vi "Lab Panel V5.22.1.vi"() -> ()   [LabVIEW 2013] (continued)
                      frame #1 {
                        n566 = local read "DISP LAB01-2"() -> (w843:T4)
                        n567 = stacked-sequence {
                          tunnel: "LAB01-2" -> [w845 w847]
                          frame #0 {
                            n568 = call "sub vi - defrag tdms v1.vi"("panel id"=w845) -> ("error out"=w844:errorcluster)  [unwired: 10 in]
                            n569 = local write "data file error"(w844) -> ()
                          }
                          frame #1 {
                            n570 = call "Save data file (stop) v3.vi"("panel id"=w847) -> ("network file save error"=w846:errorcluster)  [unwired: 9 in, 1 out]
                            n571 = local write "RESULT LAB01-2"(FALSE) -> ()
                            n572 = local write "data file error"(w846) -> ()
                          }
                        }
                        n573 = Bundle(cluster=w843, "STATUS"="STOP") -> (w841:T4)  [unwired: 2 in]
                        n574 = local write "DISP LAB01-2"(w841) -> ()
                      }
                    }
                  }
                  frame True {
                    n575 = local read "SIG LAB01-2"() -> (w850:T2)
                    n576 = stacked-sequence {
                      seq-local: [w861 _] -> [_ w865]
                      tunnel: w859 -> [_ w875]
                      tunnel: w858 -> [_ w874]
                      tunnel: w857 -> [_ w873]
                      tunnel: w856 -> [_ w872]
                      tunnel: w855 -> [_ w871]
                      tunnel: [_ w870] -> w854
                      tunnel: w853 -> [_ w869]
                      tunnel: w852 -> [_ w868]
                      tunnel: w851 -> [_ w867]
                      tunnel: w850 -> [w860 w866]
                      tunnel: w849 -> [_ w864]
                      frame #0 {
                        n577 = Unbundle(w860) -> ("AMPS"=w863:dbl)  [unwired: 4 out]
                        n578 = call "Check For Amps on v1.vi"("ID"="LAB01-2", "amps"=w863) -> ("amps"=w861:bool)  [unwired: 9 in]
                      }
                      frame #1 {
                        n579 = case shown="True" w865 {
                          tunnel: w875 -> [_ w888]
                          tunnel: w874 -> [_ w887]
                          tunnel: w873 -> [_ w886]
                          tunnel: w872 -> [_ w885]
                          tunnel: w871 -> [_ w884]
                          tunnel: [errorcluster {"status"=FALSE, "code"=0, "source"=""} ("error out") w883] -> w870
                          tunnel: w869 -> [_ w882]
                          tunnel: w868 -> [_ w881]
                          tunnel: w867 -> [_ w880]
                          tunnel: w866 -> [_ w879]
                          tunnel: w864 -> [_ w878]
                          frame False {
                            w876 = FALSE
                            n580 = local write "RUN LAB01-2"(w876) -> ()
                            n581 = local write "run lab01-2"(w876) -> ()
                          }
                          frame True {
                            n582 = stacked-sequence {
                              seq-local: [w889 _ _ _ _] -> [_ w913 _ _ _]
                              tunnel: w888 -> [w894 _ _ _ _]
                              tunnel: w887 -> [w891 _ _ _ _]
                              tunnel: w886 -> [w904 _ _ _ _]
                              tunnel: w885 -> [w897 _ _ _ _]
                              tunnel: w884 -> [w892 _ _ _ _]
                              tunnel: [_ w908 _ _ _] -> w883
                              tunnel: w882 -> [_ _ _ w935 _]
                              tunnel: w881 -> [_ _ _ w934 _]
                              tunnel: w880 -> [_ _ _ w933 _]
                              tunnel: w879 -> [_ _ _ _ _]
                              tunnel: w878 -> [_ _ _ _ w948]
                              frame #0 {
                                w890 = "\\"
                                n583 = local read "SET LAB01-2"() -> (w899:T5)
                                n584 = case shown="\"CYCLE TEST\"" w904 {
                                tunnel: ["L01-2-CHART TEST-" "L01-2-CYCLE TEST-" "L01-2-T-RISE TEST-"] -> w900
                                frame "CHART TEST", Default {
                                }
                                frame "CYCLE TEST" {
                                }
                                frame "T-RISE TEST" {
                                }
                                }
                                n585 = Unbundle(w899) -> ("DESCRIPTION"=w898:string)  [unwired: 4 out]
                                n586 = Concatenate Strings(w894, "\\", w892, w890, w891, w890) -> (w901:string)
                                n587 = String To Path(string=w901) -> (path=w903:path)
                                n588 = Concatenate Strings(w901, w900, w898, "-", w897, ".tdms") -> (w889:string)
                                n589 = Create Folder(path (use dialog)=w903) -> (error out=w902:errorcluster)  [unwired: 2 in, 2 out]
                                n590 = call <vilib>:"Clear Errors.vi"("error in (no error)"=w902) -> ()  [unwired: 6 in, 1 out]
                                n591 = global write "Global 1.vi" "LAB01-2 FILE"(w889) -> ()
                              }
                              frame #1 {
                                (unwired) FALSE
                                n592 = String To Path(string=w913) -> (path=w909:path)
                                n593 = TDMS Open(6:FALSE, 10:T21."create or replace" ("operation (0:open)"), 11:w909) -> (0:w908:errorcluster, 3:→"TDMS LAB01-2":refnum<k34>)  [unwired: 4 in]
                              }
                              frame #2 {
                                n594 = local read "SET LAB01-2"() -> (w919:T5)
                                n595 = local read "TDMS LAB01-2"() -> (w930:refnum<k34>)
                                n596 = Build Array("Testers Name", "Description", "Set Test Cycles", "T-Rise minutes", "T-Rise Deg C") -> (w920:string[])
                                n597 = Unbundle(w919) -> ("NAME"=w918:string, "DESCRIPTION"=w917:string, "CYCLES"=w916:dbl, "T-RISE mins"=w915:dbl, "T-RISE deg C"=w914:dbl)
                                n598 = Number To Decimal String(number=w916) -> (decimal integer string=w929:string)  [unwired: 1 in]
                                n599 = Number To Decimal String(number=w915) -> (decimal integer string=w928:string)  [unwired: 1 in]
                                n600 = Number To Decimal String(number=w914) -> (decimal integer string=w927:string)  [unwired: 1 in]
                                n601 = Build Array(w918, w917, w929, w928, w927) -> (w926:string[])
                                n602 = TDMS Set Properties(5:w926, 7:w920, 11:w930) -> ()  [unwired: 3 in, 4 out]
                              }
                              frame #3 {
                                n603 = local read "DISP LAB01-2"() -> (w932:T4)
                                n604 = Concatenate Strings("LAB01-2  ", w935) -> (w936:string)
                                n605 = Two Button Dialog(message=w936, 1:w933, 2:w934) -> (T button?=w938:bool)
                                n606 = case shown="True" w938 {
                                tunnel: w932 -> [w945 w946]
                                tunnel: [w945 w946] -> w942
                                tunnel: [w944 w947] -> w941
                                tunnel: [w943 w947] -> w940
                                frame False {
                                n607 = Unbundle(w945) -> ("CYCLE"=w944:dbl, "MINS"=w943:dbl)  [unwired: 1 out]
                                }
                                frame True {
                                w947 = 0.0
                                }
                                }
                                n608 = Bundle(cluster=w942, "CYCLE"=w941, "MINS"=w940, "STATUS"="RUN") -> (w931:T4)
                                n609 = local write "DISP LAB01-2"(w931) -> ()
                              }
                              frame #4 {
                                n610 = local read "TEMP START LAB01-2"() -> (w950:cluster{"TL":dbl, "TN":dbl})
                                n611 = Bundle(cluster=w950, "TL"=w948, "TN"=w948) -> (w949:cluster{"TL":dbl, "TN":dbl})
                                n612 = local write "TEMP START LAB01-2"(w949) -> ()
                              }
                            }
                          }
                        }
                      }
                    }
                  }
                }
              }
              event "RUN LAB02-1": Value Change {
                n613 = event-data() -> ("NewVal"=w956:bool)  [unwired: 1 in, 5 out]
                n614 = local read "SIG LAB02-1"() -> (w952:T2)
                n615 = case shown="True" w956 {
                  tunnel: w962 -> [_ w1000]
                  tunnel: w961 -> [_ w999]
                  tunnel: w959 -> [w964 w998]
                  tunnel: w960 -> [_ w997]
                  tunnel: w958 -> [_ w996]
                  tunnel: [w963 w995] -> w957
                  tunnel: w955 -> [_ w994]
                  tunnel: w954 -> [_ w993]
                  tunnel: w953 -> [_ w992]
                  tunnel: w952 -> [_ w991]
                  tunnel: w951 -> [_ w990]
                  frame False {
                    # "stop test"
                    n616 = stacked-sequence {
                      tunnel: w964 -> [w973 _]
                      tunnel: [w965 _] -> w963
                      frame #0 {
                        n617 = local read "DISP LAB02-1"() -> (w972:T4)
                        n618 = Unbundle(w972) -> ("CYCLE"=w970:dbl, "MINS"=w971:dbl)  [unwired: 1 out]
                        n619 = case shown="\"CYCLE TEST\"" w973 {
                          tunnel: w971 -> [_ _ w980]
                          tunnel: w970 -> [w978 w979 _]
                          tunnel: [w978 w979 w980] -> w969
                          frame "CHART TEST", Default {
                          }
                          frame "CYCLE TEST" {
                          }
                          frame "T-RISE TEST" {
                          }
                        }
                        n620 = local read "TDMS LAB02-1"() -> (w977:refnum<k34>)
                        n621 = Build Array("STOPPED") -> (w974:string[])
                        n622 = Build Array(w969) -> (w968:dbl[])
                        n623 = TDMS Write(0:w977, 5:"TEST RESULT", 7:w974, 9:w968) -> (4:w966:refnum<k34>, 15:w967:errorcluster)  [unwired: 2 in, 2 out]
                        n624 = TDMS Close(8:w967, 11:w966) -> (0:w965:errorcluster)  [unwired: 1 out]
                      }
                      frame #1 {
                        n625 = local read "DISP LAB02-1"() -> (w984:T4)
                        n626 = stacked-sequence {
                          tunnel: "LAB02-1" -> [w986 w988]
                          frame #0 {
                            n627 = call "sub vi - defrag tdms v1.vi"("panel id"=w986) -> ("error out"=w985:errorcluster)  [unwired: 10 in]
                            n628 = local write "data file error"(w985) -> ()
                          }
                          frame #1 {
                            n629 = local write "RESULT LAB02-1"(FALSE) -> ()
                            n630 = call "Save data file (stop) v3.vi"("panel id"=w988) -> ("network file save error"=w987:errorcluster)  [unwired: 9 in, 1 out]
                            n631 = local write "data file error"(w987) -> ()
                          }
                        }
                        n632 = Bundle(cluster=w984, "STATUS"="STOP") -> (w982:T4)  [unwired: 2 in]
                        n633 = local write "DISP LAB02-1"(w982) -> ()
                      }
                    }
                  }
                  frame True {
                    n634 = stacked-sequence {
                      seq-local: [w1002 _] -> [_ w1006]
                      tunnel: w1000 -> [_ w1016]
                      tunnel: w999 -> [_ w1015]
                      tunnel: w998 -> [_ w1014]
                      tunnel: w997 -> [_ w1013]
                      tunnel: w996 -> [_ w1012]
                      tunnel: [_ w1011] -> w995
                      tunnel: w994 -> [_ w1010]
                      tunnel: w993 -> [_ w1009]
                      tunnel: w992 -> [_ w1008]
                      tunnel: w991 -> [w1001 w1007]
                      tunnel: w990 -> [_ w1005]
                      frame #0 {
                        n635 = Unbundle(w1001) -> ("AMPS"=w1004:dbl)  [unwired: 4 out]
                        n636 = call "Check For Amps on v1.vi"("ID"="LAB02-1", "amps"=w1004) -> ("amps"=w1002:bool)  [unwired: 9 in]
                      }
                      frame #1 {
                        n637 = case shown="True" w1006 {
                          tunnel: w1016 -> [_ w1029]
                          tunnel: w1015 -> [_ w1028]
                          tunnel: w1014 -> [_ w1027]
                          tunnel: w1013 -> [_ w1026]
                          tunnel: w1012 -> [_ w1025]
                          tunnel: [errorcluster {"status"=FALSE, "code"=0, "source"=""} ("error out") w1024] -> w1011
                          tunnel: w1010 -> [_ w1023]
                          tunnel: w1009 -> [_ w1022]
                          tunnel: w1008 -> [_ w1021]
                          tunnel: w1007 -> [_ w1020]
                          tunnel: w1005 -> [_ w1019]
                          frame False {
                            w1018 = FALSE
                            n638 = local write "RUN LAB02-1"(w1018) -> ()
                            n639 = local write "run lab02-1"(w1018) -> ()
                          }
                          frame True {
                            n640 = stacked-sequence {
                              seq-local: [w1030 _ _ _ _] -> [_ w1054 _ _ _]
                              tunnel: w1029 -> [w1035 _ _ _ _]
                              tunnel: w1028 -> [w1032 _ _ _ _]
                              tunnel: w1027 -> [w1045 _ _ _ _]
                              tunnel: w1026 -> [w1038 _ _ _ _]
                              tunnel: w1025 -> [w1033 _ _ _ _]
                              tunnel: [_ w1049 _ _ _] -> w1024
                              tunnel: w1023 -> [_ _ _ w1075 _]
                              tunnel: w1022 -> [_ _ _ w1074 _]
                              tunnel: w1021 -> [_ _ _ w1073 _]
                              tunnel: w1020 -> [_ _ _ _ _]
                              tunnel: w1019 -> [_ _ _ _ w1089]
                              frame #0 {
                                w1031 = "\\"
                                n641 = local read "SET LAB02-1"() -> (w1040:T5)
                                n642 = case shown="\"CYCLE TEST\"" w1045 {
                                tunnel: ["L02-1-CHART TEST-" "L02-1-CYCLE TEST-" "L02-1-T-RISE TEST-"] -> w1041
                                frame "CHART TEST", Default {
                                }
                                frame "CYCLE TEST" {
                                }
                                frame "T-RISE TEST" {
                                }
                                }
                                n643 = Unbundle(w1040) -> ("DESCRIPTION"=w1039:string)  [unwired: 4 out]
                                n644 = Concatenate Strings(w1035, "\\", w1033, w1031, w1032, w1031) -> (w1042:string)
                                n645 = String To Path(string=w1042) -> (path=w1044:path)
                                n646 = Concatenate Strings(w1042, w1041, w1039, "-", w1038, ".tdms") -> (w1030:string)
                                n647 = Create Folder(path (use dialog)=w1044) -> (error out=w1043:errorcluster)  [unwired: 2 in, 2 out]
                                n648 = global write "Global 1.vi" "LAB02-1 FILE"(w1030) -> ()
                                n649 = call <vilib>:"Clear Errors.vi"("error in (no error)"=w1043) -> ()  [unwired: 6 in, 1 out]
                              }
                              frame #1 {
                                (unwired) FALSE
                                n650 = String To Path(string=w1054) -> (path=w1050:path)
                                n651 = TDMS Open(6:FALSE, 10:T21."create or replace" ("operation (0:open)"), 11:w1050) -> (0:w1049:errorcluster, 3:→"TDMS LAB02-1":refnum<k34>)  [unwired: 4 in]
                              }
                              frame #2 {
                                n652 = local read "SET LAB02-1"() -> (w1060:T5)
                                n653 = local read "TDMS LAB02-1"() -> (w1071:refnum<k34>)
                                n654 = Build Array("Testers Name", "Description", "Set Test Cycles", "T-Rise minutes", "T-Rise Deg C") -> (w1061:string[])
                                n655 = Unbundle(w1060) -> ("NAME"=w1059:string, "DESCRIPTION"=w1058:string, "CYCLES"=w1057:dbl, "T-RISE mins"=w1056:dbl, "T-RISE deg C"=w1055:dbl)
                                n656 = Number To Decimal String(number=w1057) -> (decimal integer string=w1070:string)  [unwired: 1 in]
                                n657 = Number To Decimal String(number=w1056) -> (decimal integer string=w1069:string)  [unwired: 1 in]
                                n658 = Number To Decimal String(number=w1055) -> (decimal integer string=w1068:string)  [unwired: 1 in]
                                n659 = Build Array(w1059, w1058, w1070, w1069, w1068) -> (w1067:string[])
                                n660 = TDMS Set Properties(5:w1067, 7:w1061, 11:w1071) -> ()  [unwired: 3 in, 4 out]
                              }
                              frame #3 {
                                n661 = local read "DISP LAB02-1"() -> (w1076:T4)
                                n662 = Concatenate Strings("LAB02-1  ", w1075) -> (w1077:string)
                                n663 = Two Button Dialog(message=w1077, 1:w1073, 2:w1074) -> (T button?=w1079:bool)
                                n664 = case shown="True" w1079 {
                                tunnel: w1076 -> [w1086 w1087]
                                tunnel: [w1086 w1087] -> w1083
                                tunnel: [w1085 w1088] -> w1082
                                tunnel: [w1084 w1088] -> w1081
                                frame False {
                                n665 = Unbundle(w1086) -> ("CYCLE"=w1085:dbl, "MINS"=w1084:dbl)  [unwired: 1 out]
                                }
                                frame True {
                                w1088 = 0.0
                                }
                                }
                                n666 = Bundle(cluster=w1083, "CYCLE"=w1082, "MINS"=w1081, "STATUS"="RUN") -> (w1072:T4)
                                n667 = local write "DISP LAB02-1"(w1072) -> ()
                              }
                              frame #4 {
                                n668 = local read "TEMP START LAB02-1"() -> (w1091:cluster{"TL":dbl, "TN":dbl})
                                n669 = Bundle(cluster=w1091, "TL"=w1089, "TN"=w1089) -> (w1090:cluster{"TL":dbl, "TN":dbl})
                                n670 = local write "TEMP START LAB02-1"(w1090) -> ()
                              }
                            }
                          }
                        }
                      }
                    }
                  }
                }
                n671 = local write "run lab02-1"(w956) -> ()
              }
              event "RUN LAB02-2": Value Change {
                n672 = event-data() -> ("NewVal"=w1096:bool)  [unwired: 1 in, 5 out]
                n673 = local write "run lab02-2"(w1096) -> ()
                n674 = case shown="True" w1096 {
                  tunnel: w1102 -> [_ w1140]
                  tunnel: w1101 -> [_ w1139]
                  tunnel: w1099 -> [w1104 w1138]
                  tunnel: w1100 -> [_ w1137]
                  tunnel: w1098 -> [_ w1136]
                  tunnel: [w1103 w1135] -> w1097
                  tunnel: w1095 -> [_ w1134]
                  tunnel: w1094 -> [_ w1133]
                  tunnel: w1093 -> [_ w1132]
                  tunnel: w1092 -> [_ w1130]
                  frame False {
                    # "stop test"
                    n675 = stacked-sequence {
                      tunnel: w1104 -> [w1113 _]
                      tunnel: [w1105 _] -> w1103
                      frame #0 {
                        n676 = local read "DISP LAB02-2"() -> (w1112:T4)
                        n677 = Unbundle(w1112) -> ("CYCLE"=w1110:dbl, "MINS"=w1111:dbl)  [unwired: 1 out]
                        n678 = case shown="\"CYCLE TEST\"" w1113 {
                          tunnel: w1111 -> [_ _ w1120]
                          tunnel: w1110 -> [w1118 w1119 _]
                          tunnel: [w1118 w1119 w1120] -> w1109
                          frame "CHART TEST", Default {
                          }
                          frame "CYCLE TEST" {
                          }
                          frame "T-RISE TEST" {
                          }
                        }
                        n679 = local read "TDMS LAB02-2"() -> (w1117:refnum<k34>)
                        n680 = Build Array("STOPPED") -> (w1114:string[])
                        n681 = Build Array(w1109) -> (w1108:dbl[])
                        n682 = TDMS Write(0:w1117, 5:"TEST RESULT", 7:w1114, 9:w1108) -> (4:w1106:refnum<k34>, 15:w1107:errorcluster)  [unwired: 2 in, 2 out]
                        n683 = TDMS Close(8:w1107, 11:w1106) -> (0:w1105:errorcluster)  [unwired: 1 out]
                      }
                      frame #1 {
                        n684 = local read "DISP LAB02-2"() -> (w1124:T4)
                        n685 = stacked-sequence {
                          tunnel: "LAB02-2" -> [w1126 w1128]
                          frame #0 {
                            n686 = call "sub vi - defrag tdms v1.vi"("panel id"=w1126) -> ("error out"=w1125:errorcluster)  [unwired: 10 in]
                            n687 = local write "data file error"(w1125) -> ()
                          }
                          frame #1 {
                            n688 = call "Save data file (stop) v3.vi"("panel id"=w1128) -> ("network file save error"=w1127:errorcluster)  [unwired: 9 in, 1 out]
                            n689 = local write "RESULT LAB02-2"(FALSE) -> ()
                            n690 = local write "data file error"(w1127) -> ()
                          }
                        }
                        n691 = Bundle(cluster=w1124, "STATUS"="STOP") -> (w1122:T4)  [unwired: 2 in]
                        n692 = local write "DISP LAB02-2"(w1122) -> ()
                      }
                    }
                  }
                  frame True {
                    n693 = local read "SIG LAB02-2"() -> (w1131:T2)
                    n694 = stacked-sequence {
                      seq-local: [w1142 _] -> [_ w1146]
                      tunnel: w1140 -> [_ w1156]
                      tunnel: w1139 -> [_ w1155]
                      tunnel: w1138 -> [_ w1154]
                      tunnel: w1137 -> [_ w1153]
                      tunnel: w1136 -> [_ w1152]
                      tunnel: [_ w1151] -> w1135
                      tunnel: w1134 -> [_ w1150]
                      tunnel: w1133 -> [_ w1149]
                      tunnel: w1132 -> [_ w1148]
                      tunnel: w1131 -> [w1141 w1147]
                      tunnel: w1130 -> [_ w1145]
                      frame #0 {
                        n695 = Unbundle(w1141) -> ("AMPS"=w1144:dbl)  [unwired: 4 out]
                        n696 = call "Check For Amps on v1.vi"("ID"="LAB02-2", "amps"=w1144) -> ("amps"=w1142:bool)  [unwired: 9 in]
                      }
                      frame #1 {
                        n697 = case shown="True" w1146 {
                          tunnel: w1156 -> [_ w1169]
                          tunnel: w1155 -> [_ w1168]
                          tunnel: w1154 -> [_ w1167]
                          tunnel: w1153 -> [_ w1166]
                          tunnel: w1152 -> [_ w1165]
                          tunnel: [errorcluster {"status"=FALSE, "code"=0, "source"=""} ("error out") w1164] -> w1151
                          tunnel: w1150 -> [_ w1163]
                          tunnel: w1149 -> [_ w1162]
                          tunnel: w1148 -> [_ w1161]
                          tunnel: w1147 -> [_ w1160]
                          tunnel: w1145 -> [_ w1159]
                          frame False {
                            w1157 = FALSE
                            n698 = local write "RUN LAB02-2"(w1157) -> ()
                            n699 = local write "run lab02-2"(w1157) -> ()
                          }
                          frame True {
                            n700 = stacked-sequence {
                              seq-local: [w1170 _ _ _ _] -> [_ w1194 _ _ _]
                              tunnel: w1169 -> [w1175 _ _ _ _]
                              tunnel: w1168 -> [w1172 _ _ _ _]
                              tunnel: w1167 -> [w1185 _ _ _ _]
                              tunnel: w1166 -> [w1178 _ _ _ _]
                              tunnel: w1165 -> [w1173 _ _ _ _]
                              tunnel: [_ w1189 _ _ _] -> w1164
                              tunnel: w1163 -> [_ _ _ w1215 _]
                              tunnel: w1162 -> [_ _ _ w1214 _]
                              tunnel: w1161 -> [_ _ _ w1213 _]
                              tunnel: w1160 -> [_ _ _ _ _]
                              tunnel: w1159 -> [_ _ _ _ w1229]
                              frame #0 {
                                w1171 = "\\"
                                n701 = local read "SET LAB02-2"() -> (w1180:T5)
                                n702 = case shown="\"CYCLE TEST\"" w1185 {
                                tunnel: ["L02-2-CHART TEST-" "L02-2-CYCLE TEST-" "L02-2-T-RISE TEST-"] -> w1181
                                frame "CHART TEST", Default {
                                }
                                frame "CYCLE TEST" {
                                }
                                frame "T-RISE TEST" {
                                }
                                }
                                n703 = Unbundle(w1180) -> ("DESCRIPTION"=w1179:string)  [unwired: 4 out]
                                n704 = Concatenate Strings(w1175, "\\", w1173, w1171, w1172, w1171) -> (w1182:string)
                                n705 = String To Path(string=w1182) -> (path=w1184:path)
                                n706 = Concatenate Strings(w1182, w1181, w1179, "-", w1178, ".tdms") -> (w1170:string)
                                n707 = Create Folder(path (use dialog)=w1184) -> (error out=w1183:errorcluster)  [unwired: 2 in, 2 out]
                                n708 = global write "Global 1.vi" "LAB02-2 FILE"(w1170) -> ()
                                n709 = call <vilib>:"Clear Errors.vi"("error in (no error)"=w1183) -> ()  [unwired: 6 in, 1 out]
                              }
                              frame #1 {
                                (unwired) FALSE
                                n710 = String To Path(string=w1194) -> (path=w1190:path)
                                n711 = TDMS Open(6:FALSE, 10:T21."create or replace" ("operation (0:open)"), 11:w1190) -> (0:w1189:errorcluster, 3:→"TDMS LAB02-2":refnum<k34>)  [unwired: 4 in]
                              }
                              frame #2 {
                                n712 = local read "SET LAB02-2"() -> (w1200:T5)
                                n713 = local read "TDMS LAB02-2"() -> (w1211:refnum<k34>)
                                n714 = Build Array("Testers Name", "Description", "Set Test Cycles", "T-Rise minutes", "T-Rise Deg C") -> (w1201:string[])
                                n715 = Unbundle(w1200) -> ("NAME"=w1199:string, "DESCRIPTION"=w1198:string, "CYCLES"=w1197:dbl, "T-RISE mins"=w1196:dbl, "T-RISE deg C"=w1195:dbl)
                                n716 = Number To Decimal String(number=w1197) -> (decimal integer string=w1210:string)  [unwired: 1 in]
                                n717 = Number To Decimal String(number=w1196) -> (decimal integer string=w1209:string)  [unwired: 1 in]
                                n718 = Number To Decimal String(number=w1195) -> (decimal integer string=w1208:string)  [unwired: 1 in]
                                n719 = Build Array(w1199, w1198, w1210, w1209, w1208) -> (w1207:string[])
                                n720 = TDMS Set Properties(5:w1207, 7:w1201, 11:w1211) -> ()  [unwired: 3 in, 4 out]
                              }
                              frame #3 {
                                n721 = local read "DISP LAB02-2"() -> (w1216:T4)
                                n722 = Concatenate Strings("LAB02-2  ", w1215) -> (w1217:string)
                                n723 = Two Button Dialog(message=w1217, 1:w1213, 2:w1214) -> (T button?=w1219:bool)
                                n724 = case shown="True" w1219 {
                                tunnel: w1216 -> [w1226 w1227]
                                tunnel: [w1226 w1227] -> w1223
                                tunnel: [w1225 w1228] -> w1222
                                tunnel: [w1224 w1228] -> w1221
                                frame False {
                                n725 = Unbundle(w1226) -> ("CYCLE"=w1225:dbl, "MINS"=w1224:dbl)  [unwired: 1 out]
                                }
                                frame True {
                                w1228 = 0.0
                                }
                                }
                                n726 = Bundle(cluster=w1223, "CYCLE"=w1222, "MINS"=w1221, "STATUS"="RUN") -> (w1212:T4)
                                n727 = local write "DISP LAB02-2"(w1212) -> ()
                              }
                              frame #4 {
                                n728 = local read "TEMP START LAB02-2"() -> (w1231:cluster{"TL":dbl, "TN":dbl})
                                n729 = Bundle(cluster=w1231, "TL"=w1229, "TN"=w1229) -> (w1230:cluster{"TL":dbl, "TN":dbl})
                                n730 = local write "TEMP START LAB02-2"(w1230) -> ()
                              }
                            }
                          }
                        }
                      }
                    }
                  }
                }
              }
              event "RUN LAB03-1": Value Change {
                n731 = event-data() -> ("NewVal"=w1236:bool)  [unwired: 1 in, 5 out]
                n732 = local write "run lab03-1"(w1236) -> ()
                n733 = case shown="True" w1236 {
                  tunnel: w1242 -> [_ w1280]
                  tunnel: w1241 -> [_ w1279]
                  tunnel: w1239 -> [w1244 w1278]
                  tunnel: w1240 -> [_ w1277]
                  tunnel: w1238 -> [_ w1276]
                  tunnel: [w1243 w1275] -> w1237
                  tunnel: w1235 -> [_ w1274]
                  tunnel: w1234 -> [_ w1273]
                  tunnel: w1233 -> [_ w1272]
                  tunnel: w1232 -> [_ w1270]
                  frame False {
                    # "stop test"
                    n734 = stacked-sequence {
                      tunnel: w1244 -> [w1253 _]
                      tunnel: [w1245 _] -> w1243
                      frame #0 {
                        n735 = local read "DISP LAB03-1"() -> (w1252:T4)
                        n736 = Unbundle(w1252) -> ("CYCLE"=w1250:dbl, "MINS"=w1251:dbl)  [unwired: 1 out]
                        n737 = case shown="\"CYCLE TEST\"" w1253 {
                          tunnel: w1251 -> [_ _ w1260]
                          tunnel: w1250 -> [w1258 w1259 _]
                          tunnel: [w1258 w1259 w1260] -> w1249
                          frame "CHART TEST", Default {
                          }
                          frame "CYCLE TEST" {
                          }
                          frame "T-RISE TEST" {
                          }
                        }
                        n738 = local read "TDMS LAB03-1"() -> (w1257:refnum<k34>)
                        n739 = Build Array("STOPPED") -> (w1254:string[])
                        n740 = Build Array(w1249) -> (w1248:dbl[])
                        n741 = TDMS Write(0:w1257, 5:"TEST RESULT", 7:w1254, 9:w1248) -> (4:w1246:refnum<k34>, 15:w1247:errorcluster)  [unwired: 2 in, 2 out]
                        n742 = TDMS Close(8:w1247, 11:w1246) -> (0:w1245:errorcluster)  [unwired: 1 out]
                      }
                      frame #1 {
                        n743 = local read "DISP LAB03-1"() -> (w1264:T4)
                        n744 = stacked-sequence {
                          tunnel: "LAB03-1" -> [w1266 w1268]
                          frame #0 {
                            n745 = call "sub vi - defrag tdms v1.vi"("panel id"=w1266) -> ("error out"=w1265:errorcluster)  [unwired: 10 in]
                            n746 = local write "data file error"(w1265) -> ()
                          }
                          frame #1 {
                            n747 = call "Save data file (stop) v3.vi"("panel id"=w1268) -> ("network file save error"=w1267:errorcluster)  [unwired: 9 in, 1 out]
                            n748 = local write "RESULT LAB03-1"(FALSE) -> ()
                            n749 = local write "data file error"(w1267) -> ()
                          }
                        }
                        n750 = Bundle(cluster=w1264, "STATUS"="STOP") -> (w1262:T4)  [unwired: 2 in]
                        n751 = local write "DISP LAB03-1"(w1262) -> ()
                      }
                    }
                  }
                  frame True {
                    n752 = local read "SIG LAB03-1"() -> (w1271:T2)
                    n753 = stacked-sequence {
                      seq-local: [w1282 _] -> [_ w1286]
                      tunnel: w1280 -> [_ w1296]
                      tunnel: w1279 -> [_ w1295]
                      tunnel: w1278 -> [_ w1294]
                      tunnel: w1277 -> [_ w1293]
                      tunnel: w1276 -> [_ w1292]
                      tunnel: [_ w1291] -> w1275
                      tunnel: w1274 -> [_ w1290]
                      tunnel: w1273 -> [_ w1289]
                      tunnel: w1272 -> [_ w1288]
                      tunnel: w1271 -> [w1281 w1287]
                      tunnel: w1270 -> [_ w1285]
                      frame #0 {
                        n754 = Unbundle(w1281) -> ("AMPS"=w1284:dbl)  [unwired: 4 out]
                        n755 = call "Check For Amps on v1.vi"("ID"="LAB03-1", "amps"=w1284) -> ("amps"=w1282:bool)  [unwired: 9 in]
                      }
                      frame #1 {
                        n756 = case shown="True" w1286 {
                          tunnel: w1296 -> [_ w1309]
                          tunnel: w1295 -> [_ w1308]
                          tunnel: w1294 -> [_ w1307]
                          tunnel: w1293 -> [_ w1306]
                          tunnel: w1292 -> [_ w1305]
                          tunnel: [errorcluster {"status"=FALSE, "code"=0, "source"=""} ("error out") w1304] -> w1291
                          tunnel: w1290 -> [_ w1303]
                          tunnel: w1289 -> [_ w1302]
                          tunnel: w1288 -> [_ w1301]
                          tunnel: w1287 -> [_ w1300]
                          tunnel: w1285 -> [_ w1299]
                          frame False {
                            w1297 = FALSE
                            n757 = local write "RUN LAB03-1"(w1297) -> ()
                            n758 = local write "run lab03-1"(w1297) -> ()
                          }
                          frame True {
                            n759 = stacked-sequence {
                              seq-local: [w1310 _ _ _ _] -> [_ w1334 _ _ _]
                              tunnel: w1309 -> [w1315 _ _ _ _]
                              tunnel: w1308 -> [w1312 _ _ _ _]
                              tunnel: w1307 -> [w1325 _ _ _ _]
                              tunnel: w1306 -> [w1318 _ _ _ _]
                              tunnel: w1305 -> [w1313 _ _ _ _]
                              tunnel: [_ w1329 _ _ _] -> w1304
                              tunnel: w1303 -> [_ _ _ w1354 _]
                              tunnel: w1302 -> [_ _ _ w1353 _]
                              tunnel: w1301 -> [_ _ _ w1352 _]
                              tunnel: w1300 -> [_ _ _ _ _]
                              tunnel: w1299 -> [_ _ _ _ w1369]
                              frame #0 {
                                w1311 = "\\"
                                n760 = local read "SET LAB03-1"() -> (w1320:T5)
                                n761 = case shown="\"T-RISE TEST\"" w1325 {
                                tunnel: ["L03-1-CHART TEST-" "L03-1-CYCLE TEST-" "L03-1-T-RISE TEST-"] -> w1321
                                frame "CHART TEST", Default {
                                }
                                frame "CYCLE TEST" {
                                }
                                frame "T-RISE TEST" {
                                }
                                }
                                n762 = Unbundle(w1320) -> ("DESCRIPTION"=w1319:string)  [unwired: 4 out]
                                n763 = Concatenate Strings(w1315, "\\", w1313, w1311, w1312, w1311) -> (w1322:string)
                                n764 = String To Path(string=w1322) -> (path=w1324:path)
                                n765 = Concatenate Strings(w1322, w1321, w1319, "-", w1318, ".tdms") -> (w1310:string)
                                n766 = Create Folder(path (use dialog)=w1324) -> (error out=w1323:errorcluster)  [unwired: 2 in, 2 out]
                                n767 = global write "Global 1.vi" "LAB03-1 FILE"(w1310) -> ()
                                n768 = call <vilib>:"Clear Errors.vi"("error in (no error)"=w1323) -> ()  [unwired: 6 in, 1 out]
                              }
                              frame #1 {
                                (unwired) FALSE
                                n769 = String To Path(string=w1334) -> (path=w1330:path)
                                n770 = TDMS Open(6:FALSE, 10:T21."create or replace" ("operation (0:open)"), 11:w1330) -> (0:w1329:errorcluster, 3:→"TDMS LAB03-1":refnum<k34>)  [unwired: 4 in]
                              }
                              frame #2 {
                                n771 = local read "SET LAB03-1"() -> (w1340:T5)
                                n772 = local read "TDMS LAB03-1"() -> (w1351:refnum<k34>)
                                n773 = Build Array("Testers Name", "Description", "Set Test Cycles", "T-Rise minutes", "T-Rise Deg C") -> (w1341:string[])
                                n774 = Unbundle(w1340) -> ("NAME"=w1339:string, "DESCRIPTION"=w1338:string, "CYCLES"=w1337:dbl, "T-RISE mins"=w1336:dbl, "T-RISE deg C"=w1335:dbl)
                                n775 = Number To Decimal String(number=w1337) -> (decimal integer string=w1350:string)  [unwired: 1 in]
                                n776 = Number To Decimal String(number=w1336) -> (decimal integer string=w1349:string)  [unwired: 1 in]
                                n777 = Number To Decimal String(number=w1335) -> (decimal integer string=w1348:string)  [unwired: 1 in]
                                n778 = Build Array(w1339, w1338, w1350, w1349, w1348) -> (w1347:string[])
                                n779 = TDMS Set Properties(5:w1347, 7:w1341, 11:w1351) -> ()  [unwired: 3 in, 4 out]
                              }
                              frame #3 {
                                n780 = local read "DISP LAB03-1"() -> (w1356:T4)
                                n781 = Concatenate Strings("LAB03-1  ", w1354) -> (w1357:string)
                                n782 = Two Button Dialog(message=w1357, 1:w1352, 2:w1353) -> (T button?=w1359:bool)
                                n783 = case shown="True" w1359 {
                                tunnel: w1356 -> [w1366 w1367]
                                tunnel: [w1366 w1367] -> w1363
                                tunnel: [w1365 w1368] -> w1362
                                tunnel: [w1364 w1368] -> w1361
                                frame False {
                                n784 = Unbundle(w1366) -> ("CYCLE"=w1365:dbl, "MINS"=w1364:dbl)  [unwired: 1 out]
                                }
                                frame True {
                                w1368 = 0.0
                                }
                                }
                                n785 = Bundle(cluster=w1363, "CYCLE"=w1362, "MINS"=w1361, "STATUS"="RUN") -> (w1355:T4)
                                n786 = local write "DISP LAB03-1"(w1355) -> ()
                              }
                              frame #4 {
                                n787 = local read "TEMP START LAB03-1"() -> (w1371:cluster{"TL":dbl, "TN":dbl})
                                n788 = Bundle(cluster=w1371, "TL"=w1369, "TN"=w1369) -> (w1370:cluster{"TL":dbl, "TN":dbl})
                                n789 = local write "TEMP START LAB03-1"(w1370) -> ()
                              }
                            }
                          }
                        }
                      }
                    }
                  }
                }
              }
              event "RUN LAB03-2": Value Change {
                n790 = event-data() -> ("NewVal"=w1376:bool)  [unwired: 1 in, 5 out]
                n791 = local write "run lab03-2"(w1376) -> ()
                n792 = case shown="True" w1376 {
                  tunnel: w1382 -> [_ w1420]
                  tunnel: w1381 -> [_ w1419]
                  tunnel: w1379 -> [w1384 w1418]
                  tunnel: w1380 -> [_ w1417]
                  tunnel: w1378 -> [_ w1416]
                  tunnel: [w1383 w1415] -> w1377
                  tunnel: w1375 -> [_ w1414]
                  tunnel: w1374 -> [_ w1413]
                  tunnel: w1373 -> [_ w1412]
                  tunnel: w1372 -> [_ w1410]
                  frame False {
                    # "stop test"
                    n793 = stacked-sequence {
                      tunnel: w1384 -> [w1393 _]
                      tunnel: [w1385 _] -> w1383
                      frame #0 {
                        n794 = local read "DISP LAB03-2"() -> (w1392:T4)
                        n795 = Unbundle(w1392) -> ("CYCLE"=w1390:dbl, "MINS"=w1391:dbl)  [unwired: 1 out]
                        n796 = case shown="\"CYCLE TEST\"" w1393 {
                          tunnel: w1391 -> [_ _ w1400]
                          tunnel: w1390 -> [w1398 w1399 _]
                          tunnel: [w1398 w1399 w1400] -> w1389
                          frame "CHART TEST", Default {
                          }
                          frame "CYCLE TEST" {
                          }
                          frame "T-RISE TEST" {
                          }
                        }
                        n797 = local read "TDMS LAB03-2"() -> (w1397:refnum<k34>)
                        n798 = Build Array("STOPPED") -> (w1394:string[])
                        n799 = Build Array(w1389) -> (w1388:dbl[])
                        n800 = TDMS Write(0:w1397, 5:"TEST RESULT", 7:w1394, 9:w1388) -> (4:w1386:refnum<k34>, 15:w1387:errorcluster)  [unwired: 2 in, 2 out]
                        n801 = TDMS Close(8:w1387, 11:w1386) -> (0:w1385:errorcluster)  [unwired: 1 out]
                      }
                      frame #1 {
                        n802 = local read "DISP LAB03-2"() -> (w1404:T4)
                        n803 = stacked-sequence {
                          tunnel: "LAB03-2" -> [w1406 w1408]
                          frame #0 {
                            n804 = call "sub vi - defrag tdms v1.vi"("panel id"=w1406) -> ("error out"=w1405:errorcluster)  [unwired: 10 in]
                            n805 = local write "data file error"(w1405) -> ()
                          }
                          frame #1 {
                            n806 = call "Save data file (stop) v3.vi"("panel id"=w1408) -> ("network file save error"=w1407:errorcluster)  [unwired: 9 in, 1 out]
                            n807 = local write "RESULT LAB03-2"(FALSE) -> ()
                            n808 = local write "data file error"(w1407) -> ()
                          }
                        }
                        n809 = Bundle(cluster=w1404, "STATUS"="STOP") -> (w1402:T4)  [unwired: 2 in]
                        n810 = local write "DISP LAB03-2"(w1402) -> ()
                      }
                    }
                  }
                  frame True {
                    n811 = local read "SIG LAB03-2"() -> (w1411:T2)
                    n812 = stacked-sequence {
                      seq-local: [w1422 _] -> [_ w1426]
                      tunnel: w1420 -> [_ w1436]
                      tunnel: w1419 -> [_ w1435]
                      tunnel: w1418 -> [_ w1434]
                      tunnel: w1417 -> [_ w1433]
                      tunnel: w1416 -> [_ w1432]
                      tunnel: [_ w1431] -> w1415
                      tunnel: w1414 -> [_ w1430]
                      tunnel: w1413 -> [_ w1429]
                      tunnel: w1412 -> [_ w1428]
                      tunnel: w1411 -> [w1421 w1427]
                      tunnel: w1410 -> [_ w1425]
                      frame #0 {
                        n813 = Unbundle(w1421) -> ("AMPS"=w1424:dbl)  [unwired: 4 out]
                        n814 = call "Check For Amps on v1.vi"("ID"="LAB03-2", "amps"=w1424) -> ("amps"=w1422:bool)  [unwired: 9 in]
                      }
                      frame #1 {
                        n815 = case shown="True" w1426 {
                          tunnel: w1436 -> [_ w1449]
                          tunnel: w1435 -> [_ w1448]
                          tunnel: w1434 -> [_ w1447]
                          tunnel: w1433 -> [_ w1446]
                          tunnel: w1432 -> [_ w1445]
                          tunnel: [errorcluster {"status"=FALSE, "code"=0, "source"=""} ("error out") w1444] -> w1431
                          tunnel: w1430 -> [_ w1443]
                          tunnel: w1429 -> [_ w1442]
                          tunnel: w1428 -> [_ w1441]
                          tunnel: w1427 -> [_ w1440]
                          tunnel: w1425 -> [_ w1439]
                          frame False {
                            w1437 = FALSE
                            n816 = local write "RUN LAB03-2"(w1437) -> ()
                            n817 = local write "run lab03-2"(w1437) -> ()
                          }
                          frame True {
                            n818 = stacked-sequence {
                              seq-local: [w1450 _ _ _ _] -> [_ w1474 _ _ _]
                              tunnel: w1449 -> [w1455 _ _ _ _]
                              tunnel: w1448 -> [w1452 _ _ _ _]
                              tunnel: w1447 -> [w1465 _ _ _ _]
                              tunnel: w1446 -> [w1458 _ _ _ _]
                              tunnel: w1445 -> [w1453 _ _ _ _]
                              tunnel: [_ w1469 _ _ _] -> w1444
                              tunnel: w1443 -> [_ _ _ w1495 _]
                              tunnel: w1442 -> [_ _ _ w1494 _]
                              tunnel: w1441 -> [_ _ _ w1493 _]
                              tunnel: w1440 -> [_ _ _ _ _]
                              tunnel: w1439 -> [_ _ _ _ w1509]
                              frame #0 {
                                w1451 = "\\"
                                n819 = local read "SET LAB03-2"() -> (w1460:T5)
                                n820 = case shown="\"T-RISE TEST\"" w1465 {
                                tunnel: ["L03-2-CHART TEST-" "L03-2-CYCLE TEST-" "L03-2-T-RISE TEST-"] -> w1461
                                frame "CHART TEST", Default {
                                }
                                frame "CYCLE TEST" {
                                }
                                frame "T-RISE TEST" {
                                }
                                }
                                n821 = Unbundle(w1460) -> ("DESCRIPTION"=w1459:string)  [unwired: 4 out]
                                n822 = Concatenate Strings(w1455, "\\", w1453, w1451, w1452, w1451) -> (w1462:string)
                                n823 = String To Path(string=w1462) -> (path=w1464:path)
                                n824 = Concatenate Strings(w1462, w1461, w1459, "-", w1458, ".tdms") -> (w1450:string)
                                n825 = Create Folder(path (use dialog)=w1464) -> (error out=w1463:errorcluster)  [unwired: 2 in, 2 out]
                                n826 = global write "Global 1.vi" "LAB03-2 FILE"(w1450) -> ()
                                n827 = call <vilib>:"Clear Errors.vi"("error in (no error)"=w1463) -> ()  [unwired: 6 in, 1 out]
                              }
                              frame #1 {
                                (unwired) FALSE
                                n828 = String To Path(string=w1474) -> (path=w1470:path)
                                n829 = TDMS Open(6:FALSE, 10:T21."create or replace" ("operation (0:open)"), 11:w1470) -> (0:w1469:errorcluster, 3:→"TDMS LAB03-2":refnum<k34>)  [unwired: 4 in]
                              }
                              frame #2 {
                                n830 = local read "SET LAB03-2"() -> (w1480:T5)
                                n831 = local read "TDMS LAB03-2"() -> (w1491:refnum<k34>)
                                n832 = Build Array("Testers Name", "Description", "Set Test Cycles", "T-Rise minutes", "T-Rise Deg C") -> (w1481:string[])
                                n833 = Unbundle(w1480) -> ("NAME"=w1479:string, "DESCRIPTION"=w1478:string, "CYCLES"=w1477:dbl, "T-RISE mins"=w1476:dbl, "T-RISE deg C"=w1475:dbl)
                                n834 = Number To Decimal String(number=w1477) -> (decimal integer string=w1490:string)  [unwired: 1 in]
                                n835 = Number To Decimal String(number=w1476) -> (decimal integer string=w1489:string)  [unwired: 1 in]
